vi "Test.vi"() -> ()   [LabVIEW 2016]
uses:
  <vilib>/Modbus/master/Create Master Instance (Serial).vi
  <vilib>/Modbus/master/Modbus Master.lvclass
panel:
  out "register values":u16[](array[numeric])
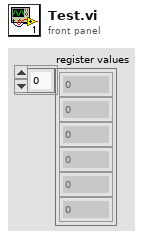
[diagram p1: front panel]
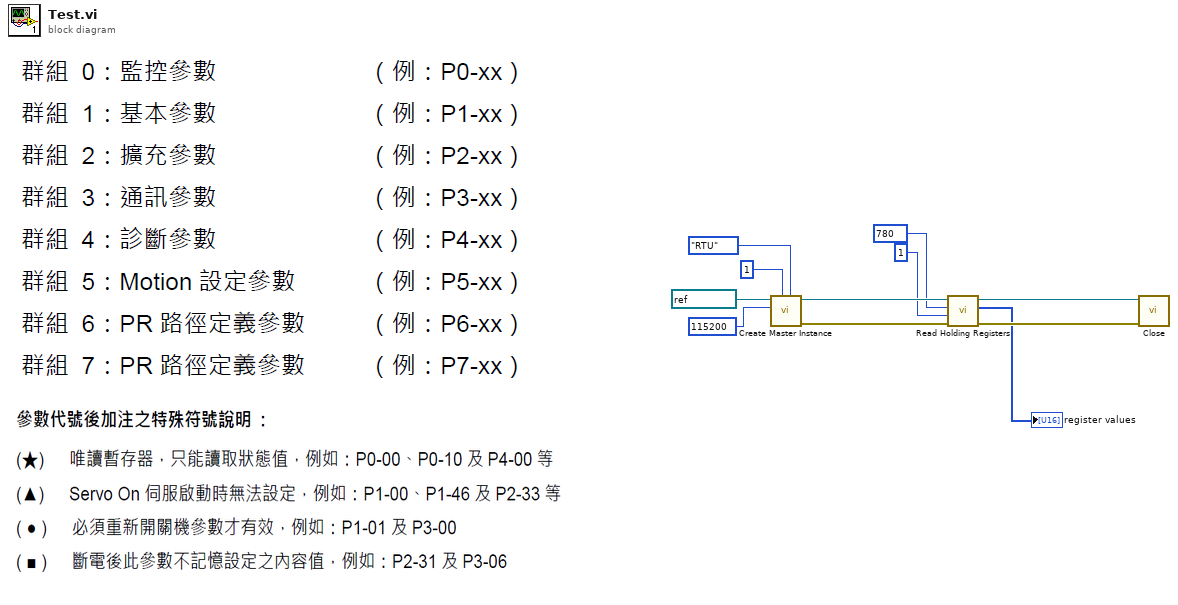
[diagram p0: block diagram]
diagram:
  n1 = call-poly <vilib>:"Create Master Instance.vi"("serial type"=enum16{"RTU", "ASCII"}."RTU", "unit ID"=u8 1, "baud rate (9600)"=u32 115200, "VISA resource name"=refnum<visa-resource-name> "COM6") -> ("error out"=w6:errorcluster, "serial master instance"=w7:refnum<class "Modbus Master.lvclass">)  [unwired: 6 in]
  n2 = call-dynamic "Read Holding Registers.vi"("error in (no error)"=w6, "number of holding registers"=u16 1, "starting address"=u16 780, "Modbus master in"=w7) -> ("error out"=w5:errorcluster, "register values"=→"register values":u16[], "Modbus master out"=w4:refnum<class "Modbus Master.lvclass">)  [unwired: 5 in]
  n3 = call-dynamic "Close.vi"("error in (no error)"=w5, "Modbus master in"=w4) -> ()  [unwired: 9 in, 1 out]
